vi "RT Driver_Watchdog.vi"(8 "error in (no error)":errorcluster, 9 "Inputs In":dbl[](array[numeric]), 11 "Outputs In":dbl[](array[numeric])) -> (0 "error out":errorcluster, 3 "Outputs Out":dbl[](array[numeric]))   [LabVIEW 2013, in "SNTP Light Custom Device Engine.lvlib"]
uses:
  SNTP Light Custom Device Engine.lvlib
  <vilib>/NI_Real-Time Target Support.lvlib
  <vilib>/NI Veristand/Custom Device Tools/Custom Device Utility Library/Custom Device Utility Library.lvlib
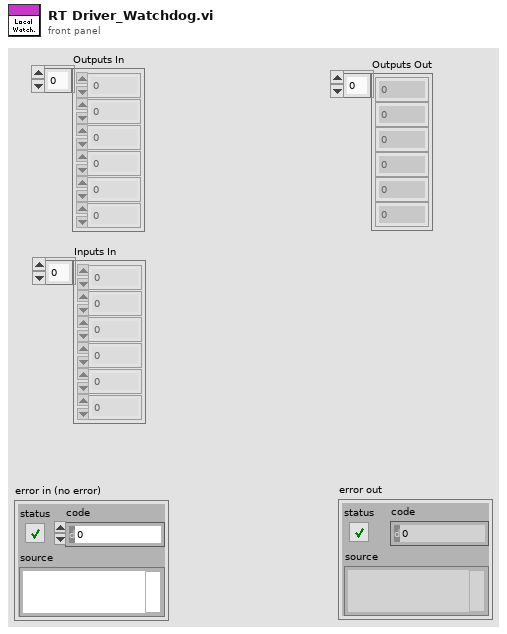
[diagram p1: front panel]
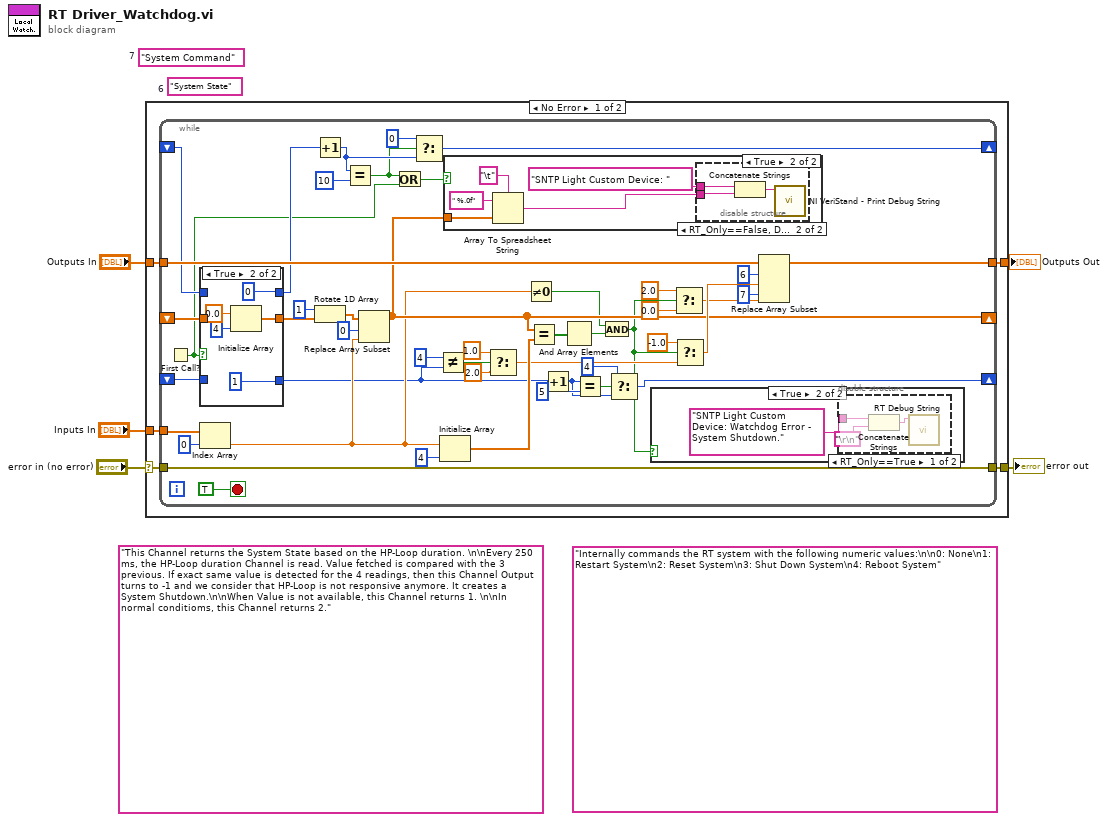
[diagram p0: block diagram]
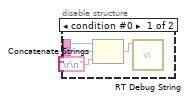
[diagram p3: hidden frame]
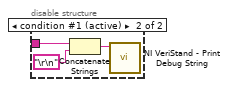
[diagram p5: hidden frame]
diagram:
  (unwired) "Internally commands the RT system with the following numeric values:\n\n0: None\n1: Restart System\n2: Reset System\n3: Shut Down System\n4: Reboot System" ("Description")
  (unwired) "This Channel returns the System State based on the HP-Loop duration. \n\nEvery 250 ms, the HP-Loop duration Channel is read. Value fetched is compared with the 3 previous. If exact same value is detected for the 4 readings, then this Channel Output turns to -1 and we consider that HP-Loop is not responsive anymore. It creates a System Shutdown.\n\nWhen Value is not available, this Channel returns 1. \n\nIn normal conditioms, this Channel returns 2." ("Description")
  (unwired) "System Command"  # 7
  (unwired) "System State"  # 6
  n1 = case shown="No Error" "error in (no error)" {
    selector: "error in (no error)" -> [w10 w86]
    tunnel: [w7 w86] -> w4
    tunnel: "Outputs In" -> [w9 w85]
    tunnel: [w6 w85] -> w2
    tunnel: "Inputs In" -> [w8 _]
    frame No Error {
      n2 = while {
        tunnel: w10 -> [w53]
        tunnel: w9 -> [w42]
        tunnel: w8 -> [w56]
        shift-right: [w24] -> _
        shift-left: _ -> [w54]
        tunnel: [w53] -> w7
        shift-right: [w11] -> _
        shift-left: _ -> [w52]
        tunnel: [w39] -> w6
        shift-right: [w25] -> _
        shift-left: _ -> [w30]
        stop <- TRUE stop-if-true
        n3 = First Call?() -> (First Call?: T/F=w21:bool)
        n4 = case shown="True" w21 {
          tunnel: [w79 w82] -> w46
          tunnel: w54 -> [w79 _]
          tunnel: [w78 u8 1] -> w16
          tunnel: w52 -> [w78 _]
          tunnel: [w77 0] -> w29
          tunnel: w30 -> [w77 _]
          frame False {
          }
          frame True {
            n5 = Initialize Array(0.0, 4 ("dimension size")) -> (w82:dbl[])
          }
        }
        n6 = Index Array(array=w56, index=0) -> (element=w17:dbl)
        n7 = Increment(x=w29) -> (x+1=w27:i32)
        n8 = Rotate 1D Array(1:w46, 2:1 ("n")) -> (0:w37:dbl[])
        n9 = Equal?(x=w27, y=10) -> (x = y?=w22:bool)
        n10 = Replace Array Subset(array=w37, new element=w17, index=0) -> (w24:dbl[])
        n11 = Or(x=w22, y=w21) -> (x .or. y?=w23:bool)
        n12 = Select(t=0, s=w22, f=w27) -> (s? t:f=w25:i32)
        n13 = Not Equal?(x=u8 4, y=w16) -> (x != y?=w50:bool)
        n14 = Initialize Array(w17, 4 ("dimension size")) -> (w44:dbl[])
        n15 = case shown="True" w23 {
          tunnel: w24 -> [_ w61]
          frame False {
          }
          frame True {
            n16 = Array To Spreadsheet String(delimiter (Tab)="\t", array=w61, 3:" %.0f" ("format string")) -> (spreadsheet string=w58:string)
            n17 = disable-structure shown="RT_Only==False, Default" {
              disable-tunnel: "SNTP Light Custom Device: " -> [w66 w68]
              disable-tunnel: w58 -> [w63 w67]
              frame condition #0 {
                n18 = Concatenate Strings(w66, w63, "\r\n") -> (w65:string)
                n19 = call <vilib>:"RT Debug String.vi"("String to write"=w65) -> ()  [unwired: 10 in, 1 out]
              }
              frame condition #1 (active) {
                n20 = Concatenate Strings(w68, w67) -> (w69:string)
                n21 = call <vilib>:"NI VeriStand - Print Debug String.vi"("Message"=w69) -> ()  [unwired: 10 in, 1 out]
              }
            }
          }
        }
        n22 = Select(t=1.0, s=w50, f=2.0) -> (s? t:f=w43:dbl)
        n23 = Not Equal To 0?(x=w17) -> (x != 0?=w18:bool)
        n24 = Equal?(x=w24, y=w44) -> (x = y?=w47:bool[])
        n25 = Increment(x=w16) -> (x+1=w12:u8)
        n26 = And Array Elements(Boolean array=w47) -> (logical AND=w20:bool)
        n27 = Equal?(x=w12, y=u8 5) -> (x = y?=w14:bool)
        n28 = And(x=w18, y=w20) -> (x .and. y?=w19:bool)
        n29 = Select(t=u8 4, s=w14, f=w12) -> (s? t:f=w11:u8)
        n30 = case shown="True" w19 {
          frame False {
          }
          frame True {
            n31 = disable-structure shown="RT_Only==True" {
              disable-tunnel: "SNTP Light Custom Device: Watchdog Error - System Shutdown." -> [w73 w74]
              frame condition #0 {
                n32 = Concatenate Strings(w73, "\r\n") -> (w72:string)
                n33 = call <vilib>:"RT Debug String.vi"("String to write"=w72) -> ()  [unwired: 10 in, 1 out]
              }
              frame condition #1 (active) {
                n34 = Concatenate Strings(w74, "\r\n") -> (w76:string)
                n35 = call <vilib>:"NI VeriStand - Print Debug String.vi"("Message"=w76) -> ()  [unwired: 10 in, 1 out]
              }
            }
          }
        }
        n36 = Select(t=2.0, s=w19, f=0.0) -> (s? t:f=w33:dbl)
        n37 = Select(t=-1.0, s=w19, f=w43) -> (s? t:f=w40:dbl)
        n38 = Replace Array Subset(array=w42, new element #1=w40, index #1=6 ("index"), new element #2=w33, index #2=7 ("index")) -> (w39:dbl[])
      }
    }
    frame Error {
    }
  }
  "error out" <- w4
  "Outputs Out" <- w2
